vi "Intensity Graph Histogram Control.vi"(8 "error in (no error)":errorcluster, 9 "lock to bin edges":bool, 10 "# std deviations for histogram width":dbl, 11 "graph_utilities in":refnum<class "graph_utilities.lvclass">) -> (0 "error out":errorcluster, 1 "Maximum":dbl, 2 "Minimum":dbl, 3 "graph_utilities out":refnum<class "graph_utilities.lvclass">)   [LabVIEW 2019, in "graph_utilities.lvclass"]
doc: "Phil's Histogram Control. Use a histogram to set your Intensity graph Z scale by easily spotting where most of your data lies."
uses:
  graph_utilities.lvclass
  graph_utilities.lvclass/graph_utilities.ctl
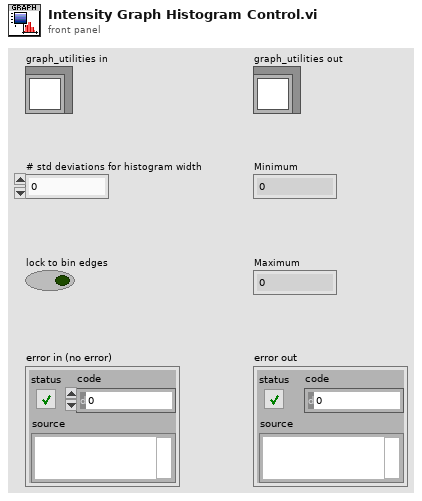
[diagram p1: front panel]
types:
  T1 = cluster{"X Values":dbl[], "Histogram: h(x)":i32[]}
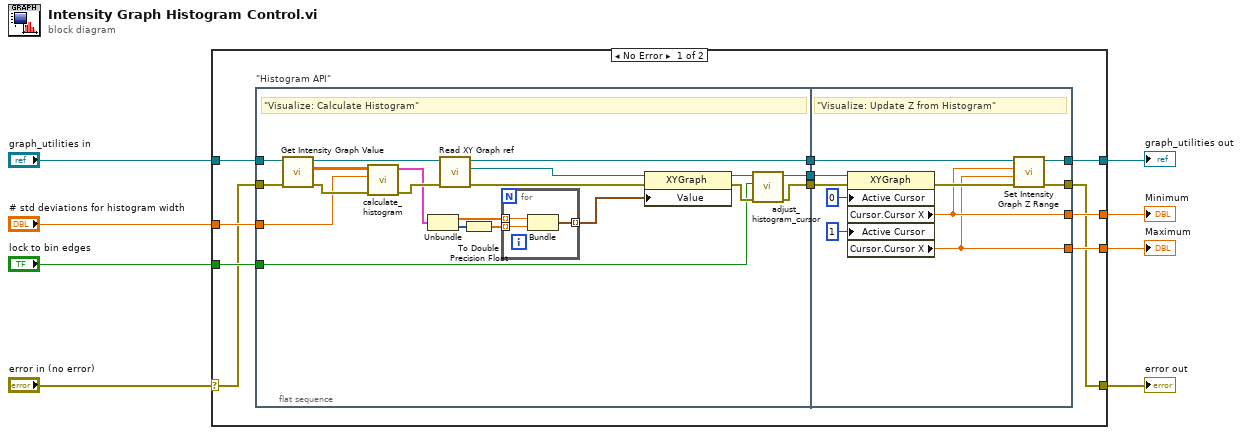
[diagram p0: block diagram]
diagram:
  n1 = case shown="No Error" "error in (no error)" {
    selector: "error in (no error)" -> [w9 w54]
    tunnel: "graph_utilities in" -> [w16 w53]
    tunnel: "# std deviations for histogram width" -> [w15 _]
    tunnel: "lock to bin edges" -> [w14 _]
    tunnel: [w13 _] -> w4
    tunnel: [w12 _] -> w5
    tunnel: [w11 w53] -> w6
    tunnel: [w10 w54] -> w7
    frame No Error {
      n2 = flat-sequence "\"Histogram API\"" {
        tunnel: [w39] -> w19
        tunnel: w9 -> [w36]
        tunnel: w16 -> [w37]
        tunnel: w15 -> [w25]
        tunnel: w14 -> [w34]
        tunnel: [w27] -> w18
        tunnel: [w32] -> w17
        tunnel: w19 -> [w50]
        tunnel: w18 -> [w49]
        tunnel: [w47] -> w10
        tunnel: w17 -> [w46]
        tunnel: [w45] -> w12
        tunnel: [w44] -> w13
        tunnel: [w43] -> w11
        frame #0 {
          # "\"Visualize: Calculate Histogram\""
          n3 = call "Get Intensity Graph Value.vi"("error in (no error)"=w36, "graph_utilities in"=w37) -> ("error out"=w26:errorcluster, "Value"=w35:dbl[][], "graph_utilities out"=w30:refnum<class "graph_utilities.lvclass">)  [unwired: 7 in]
          n4 = call "calculate_histogram.vi"("error in (no error)"=w26, "# std deviations for histogram width [1]"=w25, "Intensity Graph"=w35) -> ("error out"=w28:errorcluster, "Histogram Graph"=w24:T1)  [unwired: 5 in, 2 out]
          n5 = Unbundle(w24) -> ("X Values"=w22:dbl[], "Histogram: h(x)"=w23:i32[])
          n6 = call "Read XY Graph ref.vi"("error in (no error)"=w28, "graph_utilities in"=w30) -> ("error out"=w29:errorcluster, "XY Graph"=w31:refnum<vi>, "graph_utilities out"=w27:refnum<class "graph_utilities.lvclass">)  [unwired: 6 in, 1 out]
          n7 = To Double Precision Float(number=w23) -> (double precision float=w21:dbl[])
          n8 = for {
            tunnel: w22 -> [w42] mode=indexing
            tunnel: w21 -> [w41] mode=indexing
            tunnel: [w40] -> w20 mode=indexing
            n9 = Bundle(w42, w41) -> (w40:cluster{dbl, dbl})  [unwired: 1 in]
          }
          n10 = property class="XYGraph"(reference=w31, error in=w29, "Value"=w20) -> (reference out=w33:refnum<vi>, error out=w38:errorcluster)
          n11 = call "adjust_histogram_cursor.vi"("error in (no error)"=w38, "lock to bin edges"=w34, "histogram"=w33) -> ("error out"=w39:errorcluster, "histogram out"=w32:refnum<vi>)  [unwired: 7 in]
        }
        frame #1 {
          # "\"Visualize: Update Z from Histogram\""
          n12 = property on="Property Node" class="XYGraph"(reference=w46, error in=w50, "Active Cursor"=u32 0, "Active Cursor"=u32 1) -> (error out=w48:errorcluster, "Cursor.Cursor X"=w45:dbl, "Cursor.Cursor X"=w44:dbl)  [unwired: 1 out]
          n13 = call "Set Intensity Graph Z Range.vi"("error in (no error)"=w48, "Maximum [1]"=w44, "Minimum [0]"=w45, "graph_utilities in"=w49) -> ("error out"=w47:errorcluster, "graph_utilities out"=w43:refnum<class "graph_utilities.lvclass">)  [unwired: 6 in]
        }
      }
    }
    frame Error {
    }
  }
  "error out" <- w7
  "graph_utilities out" <- w6
  "Minimum" <- w5
  "Maximum" <- w4
